vi "SAPI Speak SubVI.vi"   [LabVIEW 2009, in "SAPI.TTS.lvlib"]
uses:
  SAPI.TTS.lvlib
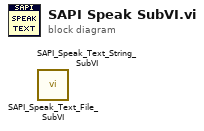
[diagram p0: block diagram]
diagram:
  n1 = call "SAPI_Speak_Text_File_SubVI.vi"() -> ()  [unwired: 10 in, 2 out]
  n2 = call "SAPI_Speak_Text_String_SubVI.vi"() -> ()  [unwired: 10 in, 2 out]
